vi "Overhead Read.vi"(8 "error in (no error)":errorcluster, 9 "Number of Blocks":i32=100, 10 "Channel Count":i32=100000, 11 "VISA resource name":refnum<visa-resource-name>) -> (0 "error out":errorcluster, 2 "Overhead Metrics":T1 {"Duration Scatter-Gather" format="%.0f µs"; "Duration N Blocks" format="%.0f µs"; "Duration 1 Block" format="%.0f µs"}, 3 "VISA resource name out":refnum<visa-resource-name>)   [LabVIEW 2016]
uses:
  Controls/Overhead Metrics.ctl
  <vilib>/Platform/TimedLoop/XDataNode/timing_clust.ctl
  <vilib>/Platform/TimedLoop/XDataNode/nitl_modes.ctl
  <vilib>/Platform/TimedLoop/XDataNode/wakeup.ctl
  Source/GE 5565PIORC/GE 5565PIORC Old.lvclass/GE 5565PIORC Old.ctl
  Source/GE 5565PIORC/VIs/Block Operations/Allocate Single Block.vi
  Source/GE 5565PIORC/VIs/DMA/DMA.Create Transfer (Single Block).vi
  Source/GE 5565PIORC/VIs/Block Operations/Allocate Multiple Blocks.vi
  Source/GE 5565PIORC/VIs/DMA/DMA.Create Transfer (Multiple Blocks).vi
  Source/GE 5565PIORC/VIs/DMA/DMA.Read Multiple.vi
  Source/GE 5565PIORC/VIs/DMA/DMA.Read Single.vi
  Source/GE 5565PIORC/VIs/Registers/Local Configuration.LAS1RR.Address Range.Get.vi
  Source/GE 5565PIORC/VIs/Registers/Local Configuration.DMACSR0.DMA Enabled.Set.vi
  Source/GE 5565PIORC/VIs/Registers/Local Configuration.INTCSR.Local DMA Interrupt Enable.Set.vi
  Source/GE 5565PIORC/VIs/Registers/Local Configuration.INTCSR.Local Interrupt Input Enable.Set.vi
  Source/GE 5565PIORC/VIs/Registers/Local Configuration.INTCSR.PCI Interrupt Enable.Set.vi
  Source/GE 5565PIORC/VIs/Binary Operations/Align to 8-byte Boundary.vi
  Source/GE 5565PIORC/VIs/Binary Operations/Align to 16-byte Boundary.vi
  Source/GE 5565PIORC/VIs/DMA/DMA.Transfer Size.vi
  Source/GE 5565PIORC/VIs/DMA/DMA.Start Transfer.vi
  Source/GE 5565PIORC/VIs/DMA/DMA.Wait for Done Interrupt Event.vi
  Source/GE 5565PIORC/VIs/Interrupts/Discard PXI Interrupt Events.vi
  Source/GE 5565PIORC/VIs/DMA/DMA.Configure.vi
  Source/GE 5565PIORC/VIs/Registers/Local Configuration.Get Register Offset.vi
  Source/GE 5565PIORC/VIs/Binary Operations/Set Bits.vi
  Source/GE 5565PIORC/VIs/Binary Operations/Set Bits U32.vi
  Source/GE 5565PIORC/VIs/Registers/Local Configuration.DMACSR0.DMA Start.Set.vi
  Source/GE 5565PIORC/VIs/Interrupts/Wait for PXI Interrupt Events.vi
  Source/GE 5565PIORC/VIs/Registers/Local Configuration.DMACSR0.DMA Clear Interrupt.Set.vi
  <vilib>/Utility/error.llb/Clear Errors.vi
  Source/GE 5565PIORC/VIs/Registers/Local Configuration.PCI Address.Set.vi
  Source/GE 5565PIORC/VIs/Registers/Local Configuration.DMADPR0.First Descriptor Address.Set.vi
  Source/GE 5565PIORC/VIs/DMA/DMA.Scatter-Gather.Link Block Descriptors.vi
  Source/GE 5565PIORC/VIs/DMA/DMA.Scatter-Gather.Commit Blocks.vi
  Source/GE 5565PIORC/VIs/Registers/Local Configuration.Local Address.Set.vi
  Source/GE 5565PIORC/VIs/Registers/Local Configuration.Transfer Size.Set.vi
  Source/GE 5565PIORC/VIs/Registers/Local Configuration.DMADPR0.Transfer Direction.Set.vi
  Source/GE 5565PIORC/VIs/Registers/Local Configuration.DMAMODE0.Scatter-Gather Enable.Set.vi
  Source/GE 5565PIORC/VIs/Binary Operations/Get Bits.vi
  Source/GE 5565PIORC/VIs/Binary Operations/Get Bits U32.vi
  Source/GE 5565PIORC/GE 5565PIORC Old.lvclass
  <vilib>/platform/TimedLoop/XDataNode/XDataNode.xnode
  <vilib>/Platform/TimedLoop/XDataNode/XDNodeRunTimeDep.lvlib
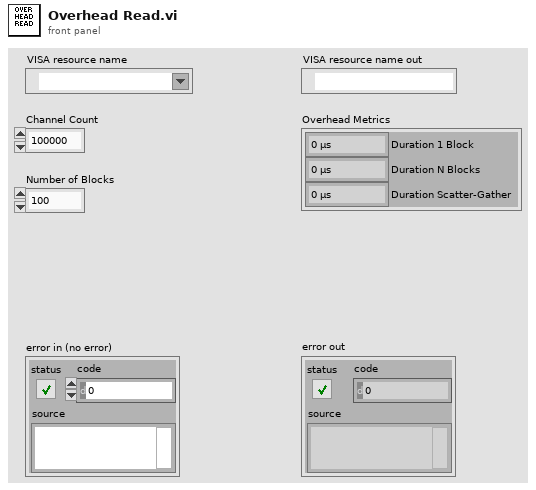
[diagram p1: front panel]
types:
  T1 = typedef "Overhead Metrics.ctl" = cluster{"Duration 1 Block":u32, "Duration N Blocks":u32, "Duration Scatter-Gather":u32}
  T2 = typedef "GE 5565PIORC Old.lvclass/DMA Block Descriptor.ctl" = cluster{"descriptor ptr (VISA)":u32, "descriptor size":u32, "descriptor ptr (aligned)":u32, "data ptr (lower)":u32, "data ptr (upper)":u32, "data size":u32, "next descriptor ptr":u32}
  T3 = typedef "GE 5565PIORC Old.lvclass/DMA Transfer Spec.ctl" = cluster{"RFM Address":u32, "Block Descriptors":T2[]}
  T4 = typedef "XDNodeRunTimeDep.lvlib/timing_clust.ctl" = cluster{"Expected End [f-1]":u64, "Actual End [f-1]":u64, "Finished Late? [f-1]":bool, "Expected End [i-1]":u64, "Actual End [i-1]":u64, "Finished Late? [i-1]":bool, "Expected Start [i]":u64, "Actual Start [i]":u64, "Expected Start [f]":u64, "Actual Start [f]":u64, "Source Name":string, "Structure Name":string, "Period":i64, "Deadline":i64, "Offset":i64, "Start":i64, "Priority":i32, "Timeout":i32, "Mode":T5, "Wakeup Reason":T6, "Error":errorcluster, "Source Type":string, "Secondary Source Type":string, "Global End Time":u64, "Global Start Time":u64, "Frame Duration":u64, "Iteration Duration":u64, "Assigned CPU":i32, "I/O Scan Engine Mode":u32}
  T5 = typedef "XDNodeRunTimeDep.lvlib/nitl_modes.ctl" = enum32{"No Change", "Process missed periods, maintain original phase", "Discard missed periods, maintain original phase", "Process missed periods, ignore original phase", "Discard missed periods, ignore original phase"}
  T6 = typedef "XDNodeRunTimeDep.lvlib/wakeup.ctl" = enum32{"Normal", "Aborted", "Asynchronous wakeup", "Timing source error", "Timed loop error", "Timeout"}
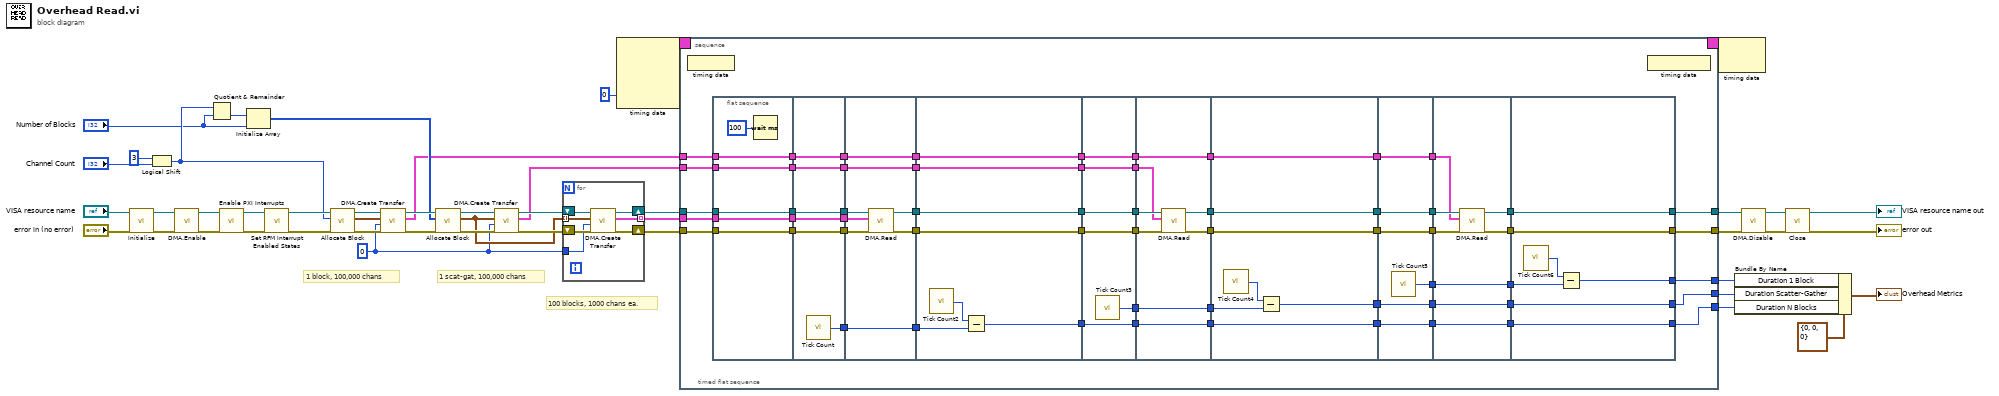
[diagram p0: block diagram]
diagram:
  w27 = u32 0 ("RFM Offset")
  # "100 blocks, 1000 chans ea."
  # "1 scat-gat, 100,000 chans"
  # "1 block, 100,000 chans"
  n1 = call "Initialize.vi"("error in (no error)"="error in (no error)", "VISA resource name"="VISA resource name") -> ("error out"=w40:errorcluster, "GE 5565PIORC"=w41:refnum<class "GE 5565PIORC Old.lvclass">)  [unwired: 8 in]
  n2 = Logical Shift(y=i16 3, x="Channel Count") -> (x << y=w8:i32)
  n3 = call "DMA.Enable.vi"("error in (no error)"=w40, "GE 5565PIORC in"=w41) -> ("error out"=w44:errorcluster, "GE 5565PIORC out"=w45:refnum<class "GE 5565PIORC Old.lvclass">)  [unwired: 8 in]
  n4 = Quotient & Remainder(x=w8, y="Number of Blocks") -> (floor(x/y)=w9:i32)  [unwired: 1 out]
  n5 = call "Enable PXI Interrupts.vi"("error in (no error)"=w44, "GE 5565PIORC in"=w45) -> ("error out"=w42:errorcluster, "GE 5565PIORC out"=w43:refnum<class "GE 5565PIORC Old.lvclass">)  [unwired: 8 in]
  n6 = Initialize Array(w9, "Number of Blocks") -> (w26:i32[])
  n7 = call "Set RFM Interrupt Enabled States.vi"("error in (no error)"=w42, "GE 5565PIORC in"=w43) -> ("error out"=w37:errorcluster, "GE 5565PIORC out"=w38:refnum<class "GE 5565PIORC Old.lvclass">)  [unwired: 8 in]
  n8 = call-poly "Allocate Block.vi"("error in (no error)"=w37, "size (bytes)"=w8, "GE 5565PIORC in"=w38) -> ("error out"=w34:errorcluster, "Block Descriptor"=w20:T2, "GE 5565PIORC out"=w36:refnum<class "GE 5565PIORC Old.lvclass">)  [unwired: 6 in]
  n9 = call-poly "DMA.Create Transfer.vi"("error in (no error)"=w34, "RFM Offset"=w27, "Block Descriptor"=w20, "GE 5565PIORC in"=w36) -> ("error out"=w33:errorcluster, "DMA Transfer Spec"=w19:T3, "GE 5565PIORC out"=w35:refnum<class "GE 5565PIORC Old.lvclass">)  [unwired: 4 in, 1 out]
  n10 = call-poly "Allocate Block.vi"("error in (no error)"=w33, "sizes (bytes)"=w26, "GE 5565PIORC in"=w35) -> ("error out"=w31:errorcluster, "Block Descriptors"=w28:T2[], "GE 5565PIORC out"=w32:refnum<class "GE 5565PIORC Old.lvclass">)  [unwired: 6 in]
  n11 = call-poly "DMA.Create Transfer.vi"("error in (no error)"=w31, "RFM Offset"=w27, "Block Descriptors"=w28, "GE 5565PIORC in"=w32) -> ("error out"=w30:errorcluster, "DMA Transfer Spec"=w18:T3, "GE 5565PIORC out"=w29:refnum<class "GE 5565PIORC Old.lvclass">)  [unwired: 4 in, 1 out]
  n12 = for {
    shift-right: [w50] -> w22
    shift-left: w29 -> [w52]
    shift-right: [w51] -> w21
    shift-left: w30 -> [w53]
    tunnel: w28 -> [w49] mode=indexing
    tunnel: w27 -> [w48]
    tunnel: [w47] -> w17 mode=indexing
    n13 = call-poly "DMA.Create Transfer.vi"("error in (no error)"=w53, "RFM Offset"=w48, "Block Descriptor"=w49, "GE 5565PIORC in"=w52) -> ("error out"=w51:errorcluster, "DMA Transfer Spec"=w47:T3, "GE 5565PIORC out"=w50:refnum<class "GE 5565PIORC Old.lvclass">)  [unwired: 4 in, 1 out]
  }
  n14 = node-c288(0 ("Processor")) -> (w25:T4)  [unwired: 3 in]
  n15 = timed-sequence {
    timing: w25 -> [_]
    timing-out: [_] -> w24
    tunnel: w22 -> [w63]
    tunnel: w21 -> [w62]
    tunnel: w19 -> [w61]
    tunnel: w18 -> [w60]
    tunnel: w17 -> [w59]
    tunnel: [w58] -> w14
    tunnel: [w57] -> w13
    tunnel: [w56] -> w4
    tunnel: [w55] -> w3
    tunnel: [w54] -> w2
    n16 = timed-flat-sequence {
      tunnel: w63 -> [w121]
      tunnel: w62 -> [w120]
      tunnel: w61 -> [w115]
      tunnel: w60 -> [w114]
      tunnel: w59 -> [w113]
      tunnel: [w77] -> w58
      tunnel: [w76] -> w57
      tunnel: [w75] -> w56
      tunnel: [w74] -> w55
      tunnel: [w64] -> w54
      n17 = node-c288() -> ()  [unwired: 1 in]
      n18 = flat-sequence {
        tunnel: w121 -> [w126]
        tunnel: w120 -> [w125]
        tunnel: [w126] -> w119
        tunnel: [w125] -> w118
        tunnel: w115 -> [w124]
        tunnel: w114 -> [w123]
        tunnel: w113 -> [w122]
        tunnel: [w124] -> w111
        tunnel: [w123] -> w109
        tunnel: [w122] -> w107
        tunnel: w119 -> [w133]
        tunnel: w118 -> [w132]
        tunnel: [w133] -> w117
        tunnel: [w132] -> w116
        tunnel: [w131] -> w112
        tunnel: w111 -> [w131]
        tunnel: [w130] -> w110
        tunnel: w109 -> [w130]
        tunnel: [w129] -> w108
        tunnel: w107 -> [w129]
        tunnel: [w128] -> w104
        tunnel: w117 -> [w141]
        tunnel: w116 -> [w140]
        tunnel: w112 -> [w134]
        tunnel: w110 -> [w135]
        tunnel: w108 -> [w139]
        tunnel: [w138] -> w106
        tunnel: [w137] -> w105
        tunnel: w104 -> [w136]
        tunnel: [w136] -> w103
        tunnel: [w135] -> w95
        tunnel: [w134] -> w92
        tunnel: w106 -> [w148]
        tunnel: w105 -> [w147]
        tunnel: w103 -> [w146]
        tunnel: [w148] -> w102
        tunnel: [w147] -> w101
        tunnel: [w144] -> w96
        tunnel: w95 -> [w144]
        tunnel: [w143] -> w93
        tunnel: w92 -> [w143]
        tunnel: [w142] -> w70
        tunnel: w102 -> [w154]
        tunnel: w101 -> [w153]
        tunnel: [w154] -> w100
        tunnel: [w153] -> w99
        tunnel: [w152] -> w98
        tunnel: [w151] -> w97
        tunnel: w96 -> [w151]
        tunnel: [w150] -> w94
        tunnel: w93 -> [w150]
        tunnel: w70 -> [w149]
        tunnel: [w149] -> w69
        tunnel: w100 -> [w160]
        tunnel: w99 -> [w161]
        tunnel: w98 -> [w162]
        tunnel: w97 -> [w159]
        tunnel: w94 -> [w156]
        tunnel: [w162] -> w91
        tunnel: [w158] -> w90
        tunnel: [w157] -> w89
        tunnel: [w156] -> w81
        tunnel: w69 -> [w155]
        tunnel: [w155] -> w68
        tunnel: w91 -> [w168]
        tunnel: w90 -> [w167]
        tunnel: w89 -> [w166]
        tunnel: [w167] -> w88
        tunnel: [w166] -> w87
        tunnel: [w165] -> w82
        tunnel: w81 -> [w165]
        tunnel: [w164] -> w71
        tunnel: w68 -> [w163]
        tunnel: [w163] -> w67
        tunnel: w88 -> [w174]
        tunnel: w87 -> [w173]
        tunnel: [w175] -> w86
        tunnel: [w174] -> w85
        tunnel: [w173] -> w84
        tunnel: [w172] -> w83
        tunnel: w82 -> [w172]
        tunnel: [w171] -> w72
        tunnel: w71 -> [w171]
        tunnel: w67 -> [w170]
        tunnel: [w170] -> w66
        tunnel: w86 -> [w183]
        tunnel: w85 -> [w182]
        tunnel: w84 -> [w181]
        tunnel: w83 -> [w178]
        tunnel: [w183] -> w80
        tunnel: [w180] -> w79
        tunnel: [w179] -> w78
        tunnel: [w177] -> w73
        tunnel: w72 -> [w177]
        tunnel: w66 -> [w176]
        tunnel: [w176] -> w65
        tunnel: [w189] -> w76
        tunnel: [w190] -> w77
        tunnel: w80 -> [w187]
        tunnel: w79 -> [w190]
        tunnel: w78 -> [w189]
        tunnel: [w186] -> w75
        tunnel: [w185] -> w74
        tunnel: w73 -> [w185]
        tunnel: w65 -> [w184]
        tunnel: [w184] -> w64
        frame #0 {
          n19 = Wait (ms)(milliseconds to wait=u32 100) -> ()  [unwired: 1 out]
        }
        frame #1 {
          n20 = call "Tick Count"() -> ("Tick Count(uSec)"=w128:u32)
        }
        frame #2 {
          n21 = call-poly "DMA.Read.vi"("error in (no error)"=w140, "DMA Transfer Specs"=w139, "GE 5565PIORC"=w141) -> ("error out"=w138:errorcluster, "GE 5565PIORC out"=w137:refnum<class "GE 5565PIORC Old.lvclass">)  [unwired: 5 in, 2 out]
        }
        frame #3 {
          n22 = call "Tick Count2"() -> ("Tick Count(uSec)"=w145:u32)
          n23 = Subtract(x=w145, y=w146) -> (x-y=w142:u32)
        }
        frame #4 {
          n24 = call "Tick Count3"() -> ("Tick Count(uSec)"=w152:u32)
        }
        frame #5 {
          n25 = call-poly "DMA.Read.vi"("error in (no error)"=w160, "DMA Transfer Spec"=w159, "GE 5565PIORC"=w161) -> ("error out"=w157:errorcluster, "GE 5565PIORC out"=w158:refnum<class "GE 5565PIORC Old.lvclass">)  [unwired: 5 in, 2 out]
        }
        frame #6 {
          n26 = call "Tick Count4"() -> ("Tick Count(uSec)"=w169:u32)
          n27 = Subtract(x=w169, y=w168) -> (x-y=w164:u32)
        }
        frame #7 {
          n28 = call "Tick Count5"() -> ("Tick Count(uSec)"=w175:u32)
        }
        frame #8 {
          n29 = call-poly "DMA.Read.vi"("error in (no error)"=w181, "DMA Transfer Spec"=w178, "GE 5565PIORC"=w182) -> ("error out"=w179:errorcluster, "GE 5565PIORC out"=w180:refnum<class "GE 5565PIORC Old.lvclass">)  [unwired: 5 in, 2 out]
        }
        frame #9 {
          n30 = call "Tick Count6"() -> ("Tick Count(uSec)"=w188:u32)
          n31 = Subtract(x=w188, y=w187) -> (x-y=w186:u32)
        }
      }
      n32 = node-c288() -> ()  [unwired: 1 out]
    }
  }
  n33 = node-c288(w24) -> ()  [unwired: 1 out]
  n34 = Bundle By Name(cluster=T1 {"Duration 1 Block"=0, "Duration N Blocks"=0, "Duration Scatter-Gather"=0} ("Overhead Metrics"), "Duration 1 Block"=w4, "Duration Scatter-Gather"=w3, "Duration N Blocks"=w2) -> (→"Overhead Metrics":T1)
  n35 = call "DMA.Disable.vi"("error in (no error)"=w13, "GE 5565PIORC in"=w14) -> ("error out"=w15:errorcluster, "GE 5565PIORC out"=w16:refnum<class "GE 5565PIORC Old.lvclass">)  [unwired: 8 in]
  n36 = call "Close.vi"("error in (no error)"=w15, "GE 5565PIORC in"=w16) -> ("error out"=→"error out":errorcluster, "VISA resource name out"=→"VISA resource name out":refnum<visa-resource-name>)  [unwired: 8 in]
